vi "getPssnAlpha.vi"(8 "error in (no error)":errorcluster, 11 "OptCtrl in":refnum<class "OptCtrl.lvclass">) -> (0 "error out":errorcluster, 2 "PSSN Alpha":dbl[](array[numeric]), 3 "OptCtrl out":refnum<class "OptCtrl.lvclass">)   [LabVIEW 2016, in "OfcFunc.lvlib" / "OptCtrl.lvclass"]
uses:
  OptCtrl.lvclass
  OptCtrl.lvclass/OptCtrl.ctl
  MatOper/MatOper.lvclass
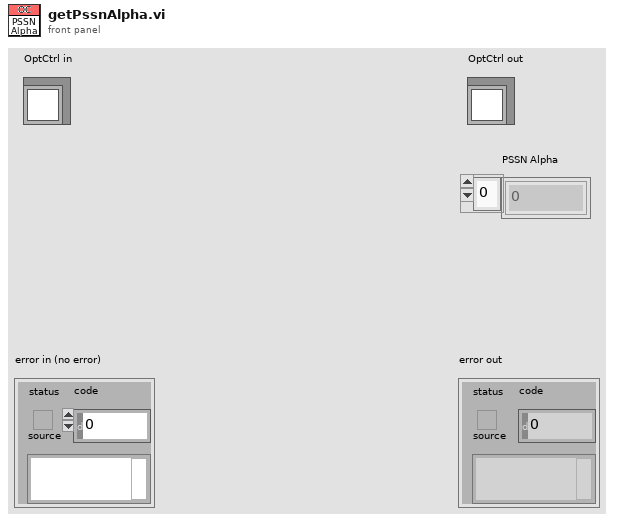
[diagram p1: front panel]
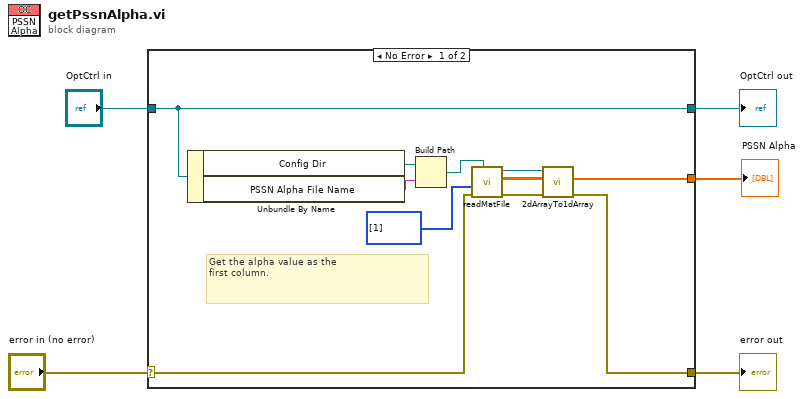
[diagram p0: block diagram]
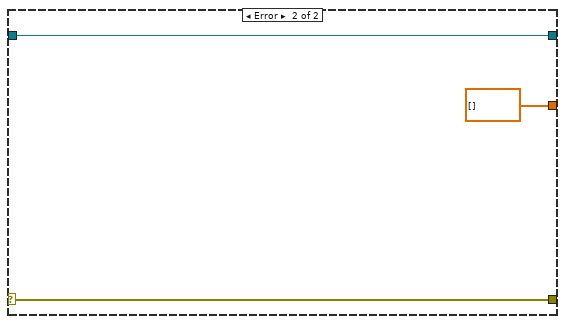
[diagram p2: hidden frame]
diagram:
  n1 = case shown="No Error" "error in (no error)" {
    selector: "error in (no error)" -> [w14 w19]
    tunnel: [w6 w19] -> w4
    tunnel: [w16 w18] -> w2
    tunnel: "OptCtrl in" -> [w16 w18]
    tunnel: [w12 dbl[] []] -> w1
    frame No Error {
      # "Get the alpha value as the \nfirst column."
      n2 = Unbundle By Name(w16) -> ("Config Dir"=w15:path, "PSSN Alpha File Name"=w13:string)
      n3 = Build Path(base path=w15, name or relative path=w13) -> (appended path=w9:path)
      n4 = call "readMatFile.vi"("Path"=w9, "error in (no error)"=w14, "Skip Col Idx"=i32[] [1]) -> ("error out"=w7:errorcluster, "Matrix"=w10:dbl[][], "MatOper out"=w8:refnum<class "MatOper.lvclass">)  [unwired: 6 in]
      n5 = call "2dArrayTo1dArray.vi"("error in (no error)"=w7, "2D Array"=w10, "MatOper in"=w8) -> ("error out"=w6:errorcluster, "1D Array"=w12:dbl[])  [unwired: 6 in, 1 out]
    }
    frame Error {
    }
  }
  "error out" <- w4
  "OptCtrl out" <- w2
  "PSSN Alpha" <- w1
